vi "Installer API Example - Main.vi"() -> ()   [LabVIEW 2017]
panel:
  in  "stop":bool
  out "counter":i32
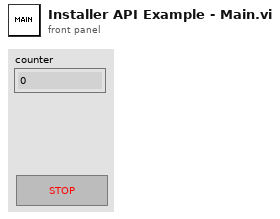
[diagram p1: front panel]
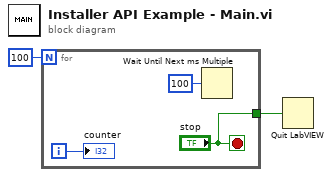
[diagram p0: block diagram]
diagram:
  n1 = for {
    N: 100 -> [_]
    tunnel: ["stop"] -> w1
    i -> [w5]
    stop <- "stop" stop-if-true
    n2 = Wait Until Next ms Multiple(millisecond multiple=u32 100) -> ()  [unwired: 1 out]
    "counter" <- w5
  }
  n3 = Quit LabVIEW(quit? (T)=w1) -> ()
